vi "rs3 create context2.vi"(8 "error in (no error)":errorcluster, 11 "api_version":i32=20000) -> (0 "error out":errorcluster, 1 "error":u64, 2 "rscontext":u64)   [LabVIEW 2017, in "libRealSense3.lvlib"]
doc: "This has to be the first call to initiate libRealSense. \nThe input is the Version Check for the libRealSense, and the output is the Context that needs to be passed to Device Count and Get Device."
uses:
  libRealSense3.lvlib
  realsense2.dll
panel:
  # "RS3 Create Context2"
  # "(C) Intel Corp.,  AGJ"
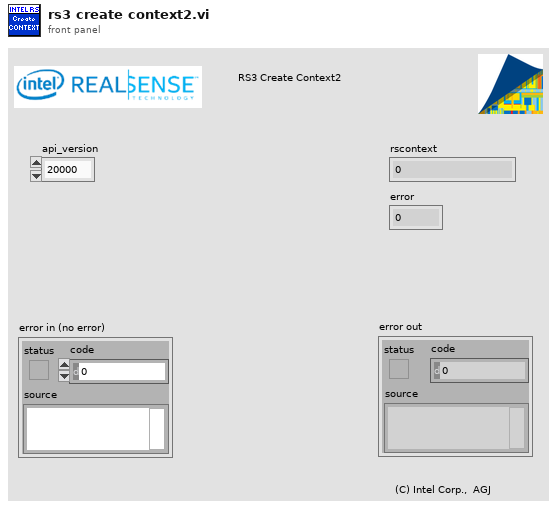
[diagram p1: front panel]
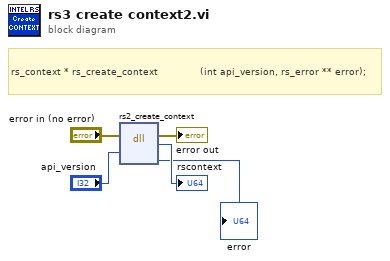
[diagram p0: block diagram]
diagram:
  # "rs_context * rs_create_context              (int api_version, rs_error ** error);"
  n1 = dll-call lib="C:/Users/agrunnet/Documents/libRealSense6/realsense2.dll" fn="rs2_create_context"(error in="error in (no error)", "api_version"="api_version") -> (error out=→"error out":errorcluster, "context"=→"rscontext":u64, "error"=→"error":u64)  [unwired: 4 in, 1 out]
